vi "Plot create flatline.vi"(9 "value":dbl, 11 "oldest,newest timestamp":u64[](array[numeric])) -> (3 "data history":T1)   [LabVIEW 2021, in "RocketPlot.lvlib"]
uses:
  RocketPlot.lvlib
  TypeDefs/plot datapoint.ctl
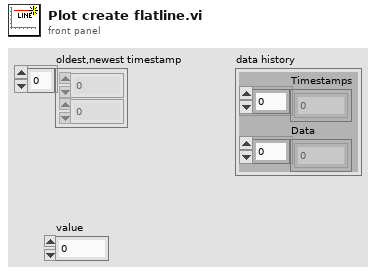
[diagram p1: front panel]
types:
  T1 = typedef "RocketPlot.lvlib/plot datapoint.ctl" = cluster{"Timestamps":u64[], "Data":dbl[]}
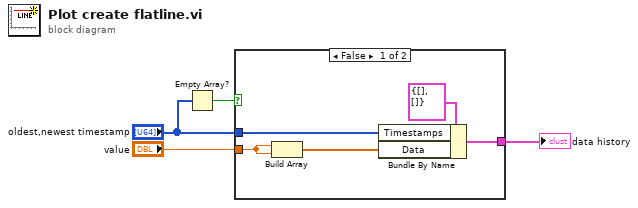
[diagram p0: block diagram]
diagram:
  n1 = Empty Array?(array="oldest,newest timestamp") -> (empty?=w2:bool)
  n2 = case shown="False" w2 {
    tunnel: "value" -> [w7 _]
    tunnel: "oldest,newest timestamp" -> [w8 _]
    tunnel: [w5 _] -> w1
    frame False {
      n3 = Build Array(w7, w7) -> (w6:dbl[])
      n4 = Bundle By Name(cluster=T1 {"Timestamps"=[], "Data"=[]} ("data history"), "Timestamps"=w8, "Data"=w6) -> (w5:T1)
    }
    frame True {
    }
  }
  "data history" <- w1
